vi "Reset Handshake - Master.vi"(0 "reset in":bool, 1 "reset handshake item":refnum<k21>) -> (4 "reset out":bool)   [LabVIEW 2018, in "Streaming FPGA.lvlib"]
doc: "Creates the reset signal for the master clock domain in a master-slave clock domain configuration.\n\nA true on the <B>reset in</B> input sets the <B>reset out</B> output to true, and this output remains true until the slave clock domain performs its reset cycle. The slave clock domain must use the <B>Reset Handshake - Slave</B> VI to receive its reset signal and to signal the completion of its reset cycle.\n\nThe resource wired to the <B>reset handshake item</B> input must be created by the <B>Reset Handshake - Create Resource</B> VI and this same resource must be wired to the <B><B>Reset Handshake - Slave</B> VI as well."
uses:
  <vilib>/rvi/DataTransferAndStorage/Container/Common/niFpgaContainerExecOnDevCompGetState.vi
  <vilib>/rvi/Emulation/niFpgaEmulationIsFPGAContextNoSignature.vi
  <vilib>/rvi/DataTransferAndStorage/Container/Common/niFpgaContainerGetUniqueNameForEmu.vi
  <vilib>/rvi/eio/common/nirviEmuReportErrorAndStop.vi
  <vilib>/rvi/Emulation/niFpgaSctlEmulationGetInTimedLoop.vi
  <vilib>/rvi/Emulation/niFpgaProcessEmulError.vi
  <vilib>/rvi/DataTransferAndStorage/Container/XNode/niFpgaContainer.xnode
  <vilib>/rvi/DataTransferAndStorage/Handshake/Emulation/niFpgaHandshakeEmulationRefIn.vi
  Streaming FPGA.lvlib
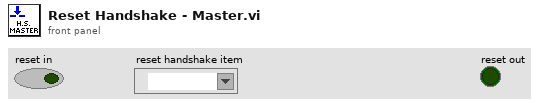
[diagram p1: front panel]
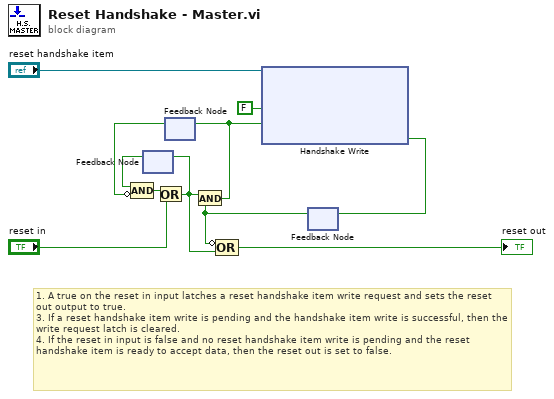
[diagram p0: block diagram]
diagram:
  # "1. A true on the reset in input latches a reset handshake item write request and sets the reset out output to true.\n3. If a reset handshake item write is pending and the handshake item write is successful, then the write request latch is cleared.\n4. If the reset in input is false and no reset handshake item write is pending and the reset handshake item is ready to accept data, then the reset out is set to false."
  n1 = feedback #1() -> (w7:bool)  [unwired: 1 in]
  n2 = feedback #2() -> (w6:bool)  [unwired: 1 in]
  n3 = Compound Arithmetic op=AND(w7, invert w6) -> (w8:bool)
  n4 = Or(x=w8, y="reset in") -> (x .or. y?=w4:bool)
  n5 = feedback-in #1(w4) -> ()
  n6 = feedback #3() -> (w3:bool)  [unwired: 1 in]
  n7 = And(x=w4, y=w3) -> (x .and. y?=w9:bool)
  n8 = feedback-in #2(w9) -> ()
  n9 = Compound Arithmetic op=OR(invert w3, w4) -> (→"reset out":bool)
  n10 = xnode "Handshake Write"("Data"=FALSE, "Input Valid"=w9, "Handshake In"="reset handshake item") -> ("Ready for Input"=w10:bool)  [unwired: 1 out]
  n11 = feedback-in #3(w10) -> ()
